vi "Text as Encoded String (UTF-8 String).vi"(9 "error in":errorcluster, 10 "Text":refnum<class "UTF-8 String.lvclass">) -> (1 "error out":errorcluster, 2 "Encoded String":T1)   [LabVIEW 2020, in "G-Unicode.lvlib"]
doc: "Converts the input string or path to a raw UTF-8 encoded LabVIEW string. Valid inputs are a UTF-8 String class, UTF-8 Path class, LabVIEW string, or LabVIEW path."
uses:
  G-Unicode.lvlib
  Types/Encoded UTF-8 String.ctl
  Types/UTF-8 String/UTF-8 String.lvclass
  Types/UTF-8 String/UTF-8 String.lvclass/UTF-8 String.ctl
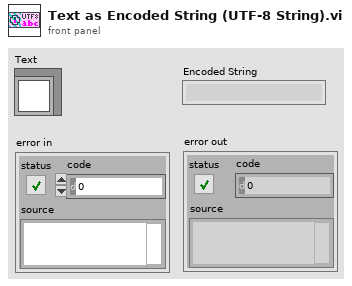
[diagram p1: front panel]
types:
  T1 = typedef "G-Unicode.lvlib/Encoded UTF-8 String.ctl" = string
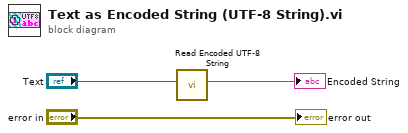
[diagram p0: block diagram]
diagram:
  n1 = call "Read Encoded UTF-8 String.vi"("UTF-8 String"="Text") -> ("Encoded UTF-8 String"=→"Encoded String":T1)  [unwired: 10 in]
  "error out" <- "error in"
